vi "Create Cluster.vi"(4 "error in":errorcluster, 6 "Cluster Definition":T1, 7 "Path":path) -> (0 "error out":errorcluster)   [LabVIEW 2025]
doc: "This VI creates a type definition (cluster) according to the provided cluster definition in the specified path. This VI sets the description and the cluster name as defined and adds the following components: numeric indicators, string controls and front panel labels."
uses:
  Cluster Definition--cluster.ctl
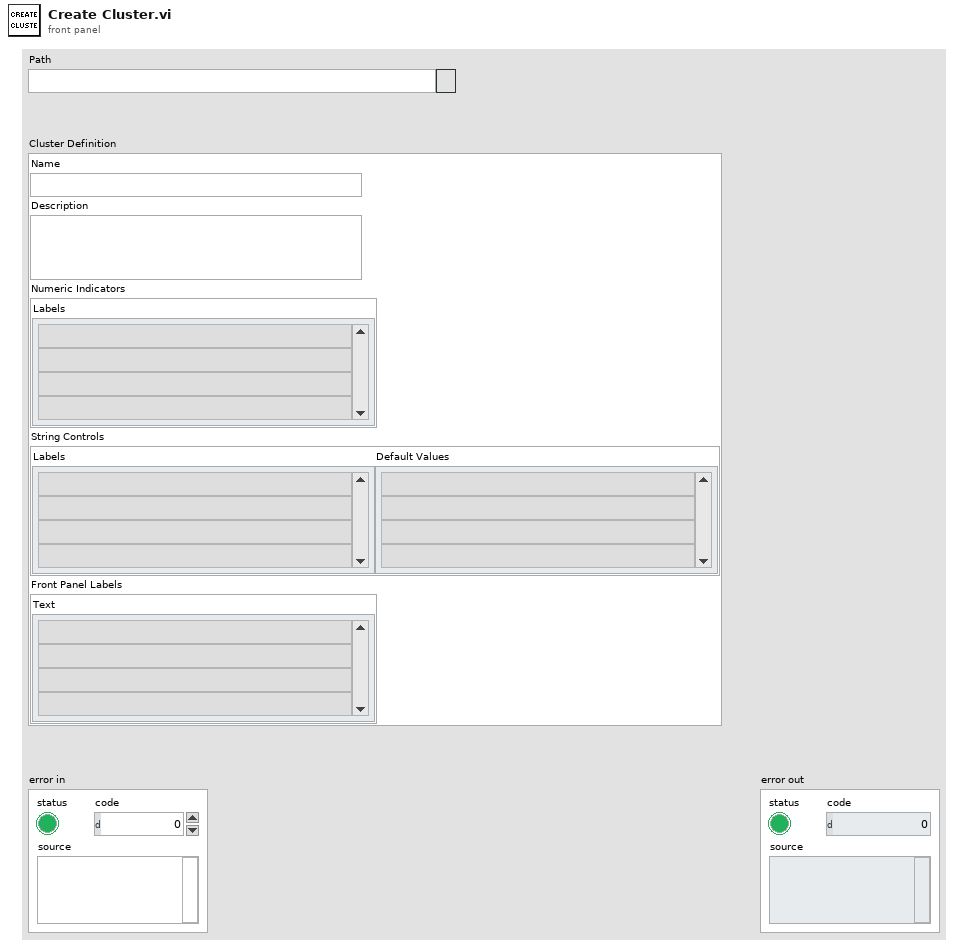
[diagram p1: front panel]
types:
  T1 = typedef "Cluster Definition--cluster.ctl" = cluster{"Name":string, "Description":string, "Numeric Indicators":cluster{"Labels":string[]}, "String Controls":cluster{"Labels":string[], "Default Values":string[]}, "Front Panel Labels":cluster{"Text":string[]}}
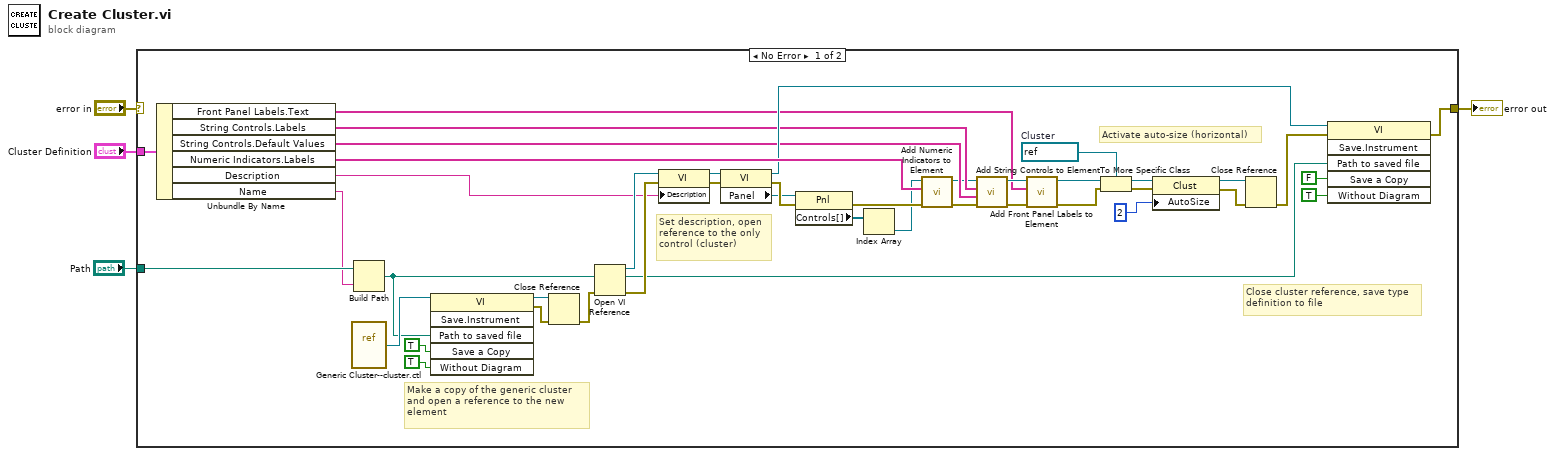
[diagram p0: block diagram]
diagram:
  n1 = case shown="No Error" "error in" {
    selector: "error in" -> [_ w46]
    tunnel: "Path" -> [w30 _]
    tunnel: "Cluster Definition" -> [w29 _]
    tunnel: [w44 w46] -> w3
    frame No Error {
      w17 = refnum<vi> refnum  # Cluster
      # "Close cluster reference, save type\ndefinition to file"
      # "Activate auto-size (horizontal)"
      # "Set description, open\nreference to the only\ncontrol (cluster)"
      # "Make a copy of the generic cluster\nand open a reference to the new\nelement"
      n2 = Unbundle By Name(w29) -> ("Front Panel Labels.Text"=w9:string[], "String Controls.Labels"=w8:string[], "String Controls.Default Values"=w7:string[], "Numeric Indicators.Labels"=w28:string[], "Description"=w11:string, "Name"=w10:string)
      n3 = vi-ref "Generic Cluster--cluster.ctl"() -> (w25:refnum<vi>)
      n4 = Build Path(base path=w30, name or relative path=w10) -> (appended path=w23:path)
      n5 = invoke class="VI" method="Save.Instrument"(reference=w25, "Path to saved file"=w23, "Save a Copy"=TRUE, "Without Diagram"=TRUE) -> (reference out=w24:refnum<vi>, error out=w42:errorcluster)  [unwired: 2 in, 4 out]
      n6 = Close Reference(reference=w24, error in (no error)=w42) -> (error out=w41:errorcluster)
      n7 = Open VI Reference(vi path=w23, error in (no error)=w41) -> (vi reference=w13:refnum<vi>, error out=w34:errorcluster)  [unwired: 4 in]
      n8 = property class="VI"(reference=w13, error in=w34, "Description"=w11) -> (reference out=w12:refnum<vi>, error out=w33:errorcluster)
      n9 = property class="VI"(reference=w12, error in=w33) -> (reference out=w19:refnum<vi>, error out=w40:errorcluster, "Panel"=w22:refnum<vi>)
      n10 = property class="Pnl"(reference=w22, error in=w40) -> (error out=w37:errorcluster, "Controls[]"=w21:refnum<vi>[])  [unwired: 1 out]
      n11 = Index Array(array=w21) -> (element=w5:refnum<vi>)  [unwired: 1 in]
      n12 = call "Add Numeric Indicators to Element.vi"("error in"=w37, "Labels"=w28, "element"=w5) -> ("error out"=w45:errorcluster, "element dup"=w6:refnum<vi>)  [unwired: 3 in]
      n13 = call "Add String Controls to Element.vi"("error in"=w45, "Values"=w7, "Labels"=w8, "element"=w6) -> ("error out"=w43:errorcluster, "element dup"=w20:refnum<vi>)  [unwired: 2 in]
      n14 = call "Add Front Panel Labels to Element.vi"("error in"=w43, "Labels"=w9, "element"=w20) -> ("error out"=w38:errorcluster, "element dup"=w18:refnum<vi>)  [unwired: 3 in]
      n15 = To More Specific Class(target class=w17, reference=w18, error in=w38) -> (specific class reference=w15:refnum<vi>, error out=w35:errorcluster)
      n16 = property class="Clust"(reference=w15, error in=w35, "AutoSize"=u32 2 ("Auto Sizing")) -> (reference out=w16:refnum<vi>, error out=w36:errorcluster)
      n17 = Close Reference(reference=w16, error in (no error)=w36) -> (error out=w39:errorcluster)
      n18 = invoke class="VI" method="Save.Instrument"(reference=w19, error in=w39, "Path to saved file"=w23, "Save a Copy"=FALSE, "Without Diagram"=TRUE) -> (error out=w44:errorcluster)  [unwired: 1 in, 5 out]
    }
    frame Error {
      # "Pass error without further action"
    }
  }
  "error out" <- w3
